vi "TIFF Find Field Info By Name.vi"(8 "error in (no error)":errorcluster, 9 "para2":cluster{}, 10 "para1":cluster{}, 11 "para0":cluster{}) -> (0 "error out":errorcluster, 2 "function return":u32, 3 "para0 out":cluster{})   [LabVIEW 2018]
doc: "LIBTIFF_DLL_IMPEXP const TIFFFieldInfo* TIFFFindFieldInfoByName(TIFF* , const char *,\n TIFFDataType);\nextern const TIFFFieldInfo* TIFFFindFieldInfoByName(TIFF* , const char *,\n TIFFDataType);"
uses:
  libtiff3.dll
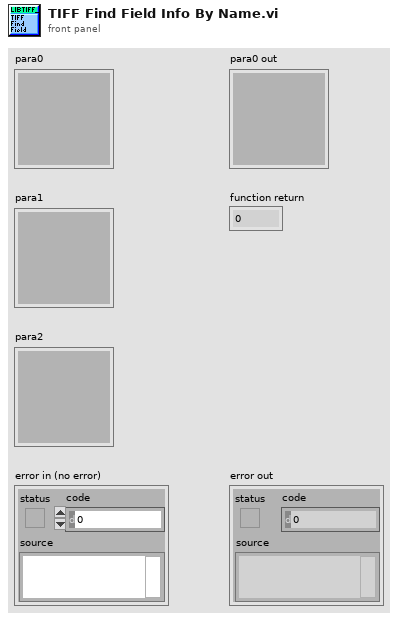
[diagram p1: front panel]
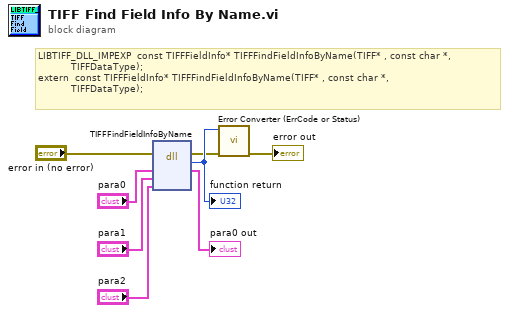
[diagram p0: block diagram]
diagram:
  # "LIBTIFF_DLL_IMPEXP  const TIFFFieldInfo* TIFFFindFieldInfoByName(TIFF* , const char *,\n\t\t\t\t\t\t     TIFFDataType);\nextern  const TIFFFieldInfo* TIFFFindFieldInfoByName(TIFF* , const char *,\n\t\t\t\t\t\t     TIFFDataType);"
  n1 = dll-call lib="C:/Users/johan/Downloads/LabVIEW software/LabVIEW software/IX-81 Software/lib/tiff/LibTiffLabview/libtiff3.*" fn="TIFFFindFieldInfoByName"(error in="error in (no error)", "para0"="para0", "para1"="para1", "para2"="para2") -> (error out=w2:errorcluster, w8:u32, "para0"=→"para0 out":cluster{})  [unwired: 4 in, 1 out]
  "function return" <- w8
  n2 = call "Error Converter (ErrCode or Status).vi"("error in (no error)"=w2, "error code"=w8) -> ("error out"=→"error out":errorcluster)  [unwired: 9 in]
